vi "chgCfgDir.vi"() -> (0 "error out":errorcluster)   [LabVIEW 2015]
panel:
  in  "Path":path=path "C:/Etion Projects/HTSTE2/StationGlobals edit - Copy"
  in  "error in (no error)":errorcluster
  in  "Application Manager":refnum<k7>(container)
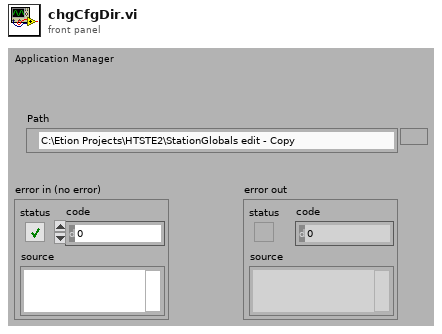
[diagram p1: front panel]
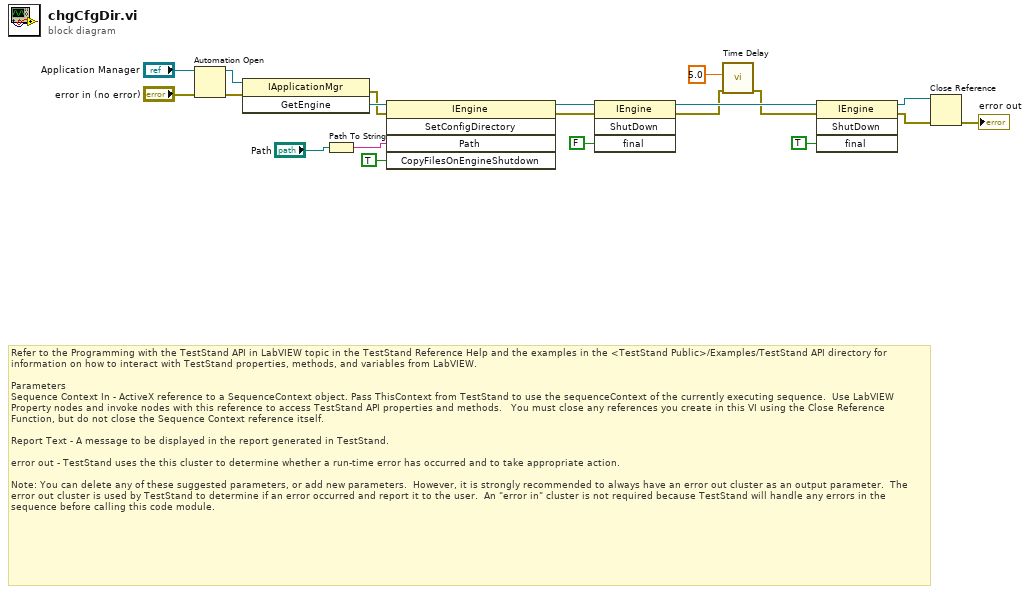
[diagram p0: block diagram]
diagram:
  # "Refer to the Programming with the TestStand API in LabVIEW topic in the TestStand Reference Help and the examples in the <TestStand Public>/Examples/TestStand API directory for information on how to interact with TestStand properties, methods, and variables from LabVIEW.\n\nParameters\nSequence Context In - ActiveX reference to a SequenceContext object. Pass ThisContext from TestStand to use the sequenceContext of the currently executing sequence.  Use LabVIEW Property nodes and invoke nodes with this reference to access TestStand API properties and methods.   You must close any references you create in this VI using the Close Reference Function, but do not close the Sequence Context reference itself.\n\nReport Text - A message to be displayed in the report generated in TestStand. \n\nerror out - TestStand uses the this cluster to determine whether a run-time error has occurred and to take appropriate action.  \n\nNote: You can delete any of these suggested parameters, or add new parameters.  However, it is strongly recommended to always have an error out cluster as an output parameter.  The error out cluster is used by TestStand to determine if an error occurred and report it to the user.  An \"error in\" cluster is not required because TestStand will handle any errors in the sequence before calling this code module."
  n1 = Automation Open(error in (no error)="error in (no error)", Automation Refnum="Application Manager") -> (Automation Refnum=w17:refnum<k7>, error out=w18:errorcluster)  [unwired: 2 in]
  n2 = invoke class="IApplicationMgr" method="GetEngine"(reference=w17, error in=w18) -> (error out=w13:errorcluster, "GetEngine"=w16:refnum<k7>)  [unwired: 1 in, 1 out]
  n3 = Path To String(path="Path") -> (string=w12:string)
  n4 = invoke class="IEngine" method="SetConfigDirectory"(reference=w16, error in=w13, "Path"=w12, "CopyFilesOnEngineShutdown"=TRUE) -> (reference out=w15:refnum<k7>, error out=w14:errorcluster)  [unwired: 1 in, 3 out]
  n5 = invoke class="IEngine" method="ShutDown"(reference=w15, error in=w14, "final"=FALSE) -> (reference out=w7:refnum<k7>, error out=w3:errorcluster)  [unwired: 1 in, 2 out]
  n6 = call "Time Delay"("error in (no error)"=w3, "Delay Time (s)"=5.0) -> ("error out"=w2:errorcluster)  [unwired: 9 in]
  n7 = invoke class="IEngine" method="ShutDown"(reference=w7, error in=w2, "final"=TRUE) -> (reference out=w5:refnum<k7>, error out=w6:errorcluster)  [unwired: 1 in, 2 out]
  n8 = Close Reference(reference=w5, error in (no error)=w6) -> (error out=→"error out":errorcluster)
